vi "Main.vi"() -> ()   [LabVIEW 2019]
doc: "The myRIO Project template acquires acceleration data from the onboard accelerometer and displays the changes of acceleration values in a waveform chart."
uses:
  <vilib>/Platform/TimedLoop/XDataNode/timing_clust.ctl
  <vilib>/Platform/TimedLoop/XDataNode/nitl_modes.ctl
  <vilib>/Platform/TimedLoop/XDataNode/wakeup.ctl
  <vilib>/myRIO/Instrument Drivers/Onboard IO/AI/typedefs/AI Reference.ctl
  <vilib>/myRIO/Common/Instrument Driver Framework/Utilities/typedefs/myRIO Generic Hardware Reference.ctl
  <vilib>/myRIO/Common/Instrument Driver Framework/Utilities/typedefs/Hardware Version Enum.ctl
  <vilib>/myRIO/Common/Instrument Driver Framework/Utilities/typedefs/myRIO v1.0 Reference.ctl
  <vilib>/myRIO/Common/Instrument Driver Framework/Utilities/typedefs/Generic FPGA Reference.ctl
  <vilib>/myRIO/Common/Instrument Driver Framework/myRIO v1.0/AI/typedefs/AI Channels List.ctl
  <vilib>/myRIO/Common/Instrument Driver Framework/myRIO v1.0/AI/typedefs/AI Channels Enum.ctl
  <vilib>/myRIO/Common/Instrument Driver Framework/Utilities/typedefs/Analog Scaling Constants List.ctl
  <vilib>/myRIO/Common/Instrument Driver Framework/Utilities/typedefs/Analog Scaling Constants.ctl
  <vilib>/userDefined/High Color/nirio_resource_hc.ctl
  <vilib>/Simulation/Shared/_Datatypes/SIM SISO Transfer Function.ctl
  <vilib>/myRIO/Instrument Drivers/Onboard IO/AO/typedefs/AO Reference.ctl
  <vilib>/myRIO/Common/Instrument Driver Framework/myRIO v1.0/AO/typedefs/AO Channels List.ctl
  <vilib>/myRIO/Common/Instrument Driver Framework/myRIO v1.0/AO/typedefs/AO Channels Enum.ctl
  <vilib>/myRIO/Common/Instrument Driver Framework/Utilities/vis/Is FPGA Ref Available.vi
  <vilib>/myRIO/Common/Instrument Driver Framework/myRIO v1.0/AI/vis/myRIO v1.1 Open AI.vi
  <vilib>/myRIO/Instrument Drivers/Onboard IO/AI/vis/Read.vi
  <vilib>/Simulation/DiscreteLinear/Implementation/NILVSim Discrete Transfer Function Direct.llb/SIM Discrete Transfer Function Diagram (SISO).vi
  <vilib>/myRIO/Common/Instrument Driver Framework/myRIO v1.0/AO/vis/myRIO v1.1 Open AO.vi
  <vilib>/myRIO/Instrument Drivers/Onboard IO/AO/vis/Write.vi
  <vilib>/myRIO/Common/Instrument Driver Framework/Utilities/vis/Validate Channels.vi
  <vilib>/myRIO/Common/Instrument Driver Framework/myRIO v1.0/AI/vis/myRIO v1.0 Reserve AI.vi
  <vilib>/Simulation/ContinuousLinear/Implementation/Shared/SIM Transfer Function Support.llb/SIM TransferFunction Normalize to Buffer.vi
  <vilib>/Simulation/DiscreteLinear/Implementation/Shared/SIM Init Discrete States.vi
  <vilib>/Simulation/DiscreteLinear/Implementation/NILVSim Discrete Transfer Function Direct.llb/SIM Transfer Function Direct core (SISO).vi
  <vilib>/myRIO/Common/Instrument Driver Framework/myRIO v1.0/AO/vis/myRIO v1.0 Reserve AO.vi
  <vilib>/myRIO/Common/Instrument Driver Framework/myRIO v1.0/AI/vis/myRIO v1.0 Build MUX Configuration AI.vi
  <vilib>/myRIO/Common/Instrument Driver Framework/myRIO v1.0/Resource Manager/vis/myRIO v1.0 Reserve Channel List.vi
  <vilib>/Simulation/ContinuousLinear/Implementation/Shared/SIM Transfer Function Support.llb/SIM TransferFunction Normalize.vi
  <vilib>/myRIO/Common/Instrument Driver Framework/myRIO v1.0/AO/vis/myRIO v1.0 Build MUX Configuration AO.vi
  <vilib>/myRIO/Common/Instrument Driver Framework/myRIO v1.0/Resource Manager/vis/myRIO v1.0 Reserve Channel.vi
  <vilib>/myRIO/Common/Instrument Driver Framework/myRIO v1.0/Resource Manager/vis/myRIO v1.0 Unreserve Channel.vi
  <vilib>/Simulation/Implementation/Shared/SIM Polynomials.llb/SIM Remove Zero Coefficients (DBL).vi
  <vilib>/myRIO/Common/Instrument Driver Framework/myRIO v1.0/Resource Manager/vis/myRIO v1.0 Build Mutex Name.vi
  <vilib>/functionblocks/Counter/Pulse Timer/Pulse Timer.vi
  <vilib>/Utility/VariantDataType/GetNumericInfo.vi
  <vilib>/Utility/error.llb/Error Cluster From Error Code.vi
  <vilib>/myRIO/Common/Instrument Driver Framework/myRIO v1.0/myRIO v1.1 Open.vi
  <vilib>/myRIO/Common/Instrument Driver Framework/myRIO v1.0/AI/vis/myRIO v1.0 Get Scaling Constants AI.vi
  <vilib>/myRIO/Common/Instrument Driver Framework/Utilities/vis/IO Manager.vi
  <vilib>/myRIO/Common/Instrument Driver Framework/Utilities/vis/Configuration Manager.vi
  <vilib>/myRIO/Common/Instrument Driver Framework/myRIO v1.0/myRIO v1.0 Close.vi
  <vilib>/myRIO/Common/Instrument Driver Framework/myRIO v1.0/AI/vis/myRIO v1.0 Read AI.vi
  <vilib>/Simulation/Implementation/Shared/SIM Polynomials.llb/SIM Divide Polynomials (DBL).vi
  <vilib>/Simulation/Implementation/Shared/SIM BuildSimErr.vi
  <vilib>/myRIO/Common/Instrument Driver Framework/myRIO v1.0/AO/vis/myRIO v1.0 Get Scaling Constants AO.vi
  <vilib>/myRIO/Common/Instrument Driver Framework/myRIO v1.0/AO/vis/myRIO v1.0 Write AO.vi
  <vilib>/platform/TimedLoop/XDataNode/XDataNode.xnode
  <vilib>/functionblocks/FB Core/FB Core.xnode
  <vilib>/myRIO/Express VI/Onboard IO/AI/AI Express VI.xnode
  <vilib>/myRIO/Instrument Drivers/Onboard IO/AI/vis/myRIO AI Open.xnode
  <vilib>/Simulation/Implementation/XNodeFramework/SimXNode/SimX.xnode
  <vilib>/myRIO/Express VI/Onboard IO/AO/AO Express VI.xnode
  <vilib>/myRIO/Instrument Drivers/Onboard IO/AO/vis/myRIO AO Open.xnode
  <vilib>/Platform/TimedLoop/XDataNode/XDNodeRunTimeDep.lvlib
  <vilib>/myRIO/Instrument Drivers/Onboard IO/AI/AI.lvlib
  <vilib>/myRIO/Instrument Drivers/Onboard IO/AO/AO.lvlib
  <vilib>/functionblocks/NI_FunctionBlock Libraries.lvlib
panel:
  out "frequecy":dbl(graph)=-0.0 caption="interrupt frequency"
  in  "interrupt time(ms)":i32=1000
  in  "Interrupt":bool
  out "sine wave":dbl(graph)=-0.0 caption="Interrupt"
  out "x[um]":dbl(graph)=2.4390249999999867
  in  "initialize z":bool
  out "right[V]":dbl=-0.00025
  out "left[V]":dbl=-0.00025
  in  "Stop EM":bool=TRUE
  out "Current Output EM":dbl(graph)=-0.0
  out "Error":errorcluster
  in  "Stop":bool
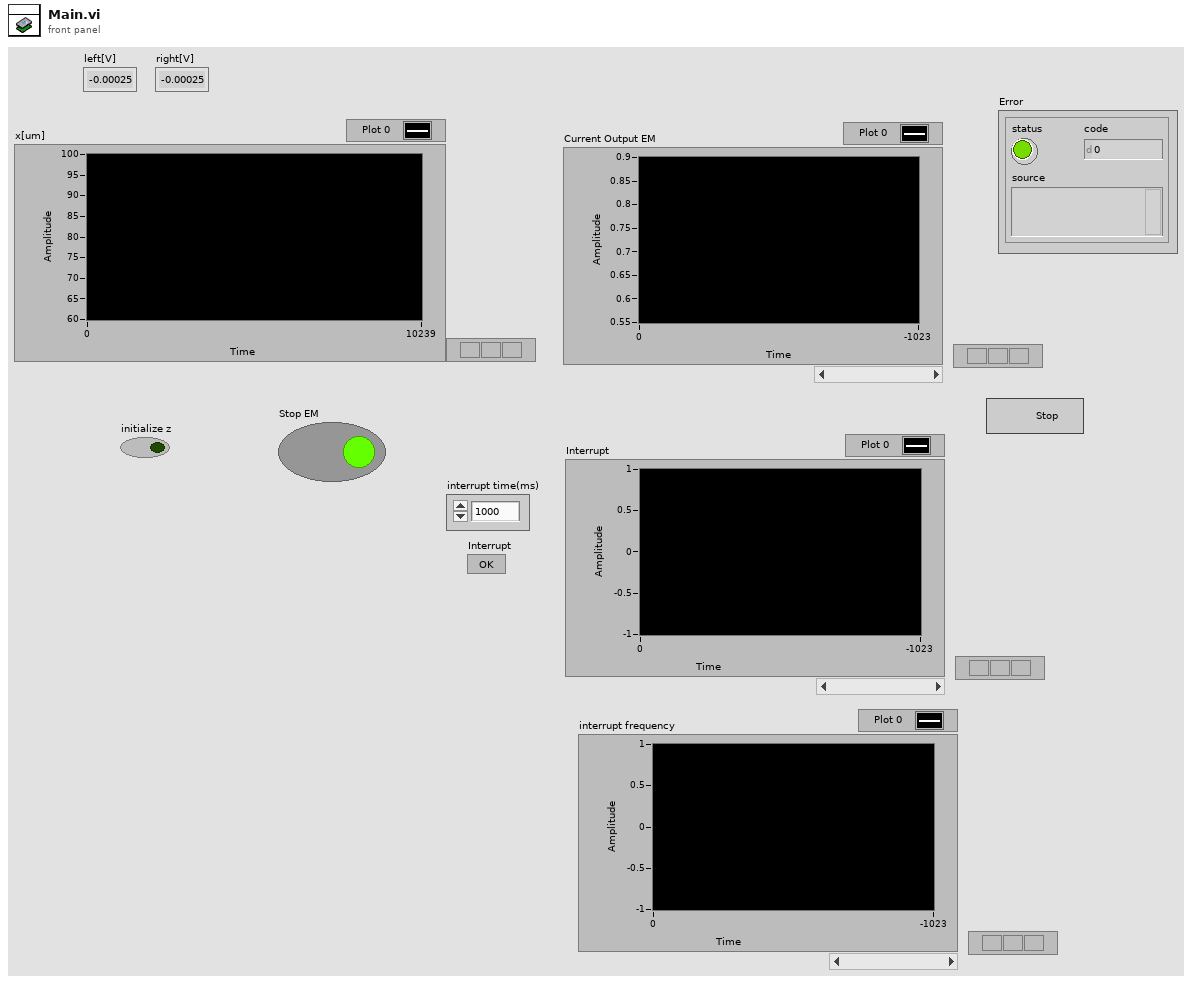
[diagram p1: front panel]
types:
  T1 = typedef "SIM SISO Transfer Function.ctl" = cluster{"Numerator":dbl[], "Denominator":dbl[]}
  T2 = typedef "AO.lvlib/AO Reference.ctl" = cluster{"myRIO Reference":T3, "AO Channel List":T7, "AO Scaling Constant List":T9}
  T3 = typedef "myRIO Generic Hardware Reference.ctl" = cluster{"myRIO Model":T4, "myRIO Hardware Reference":T5}
  T4 = typedef "Hardware Version Enum.ctl" = enum16{"Unknown", "myRIO-1900", "myRIO-1950", "roboRIO", "NI ELVIS RIO CM", "ELVIS III"}
  T5 = typedef "myRIO v1.0 Reference.ctl" = cluster{"Generic FPGA Reference":T6, "Allow multiple opens":bool}
  T6 = typedef "Generic FPGA Reference.ctl" = refnum<k20>
  T7 = typedef "AO Channels List.ctl" = T8[]
  T8 = typedef "AO Channels Enum.ctl" = enum16{"Not Connected", "AudioOut/Left", "AudioOut/Right", "C/AO0", "C/AO1", "A/AO0", "A/AO1", "B/AO0", "B/AO1"}
  T9 = typedef "Analog Scaling Constants List.ctl" = T10[]
  T10 = typedef "Analog Scaling Constants.ctl" = cluster{"LSB Weight (Volts)":dbl, "Offset (Volts)":dbl, "Signed?":bool}
  T11 = typedef "nirio_resource_hc.ctl" = tag
  T12 = typedef "AI.lvlib/AI Reference.ctl" = cluster{"myRIO Reference":T3, "AI Channels List":T13, "AI Scaling Constants List":T9}
  T13 = typedef "AI Channels List.ctl" = T14[]
  T14 = typedef "AI Channels Enum.ctl" = enum16{"Not Connected", "AudioIn/Left", "AudioIn/Right", "C/AI0", "C/AI1", "A/AI0", "A/AI1", "A/AI2", "A/AI3", "A/AI4", "A/AI5", "A/AI6", "A/AI7", "B/AI0", "B/AI1", "B/AI2", "B/AI3", "B/AI4", "B/AI5", "B/AI6", "B/AI7", "AI/AI0", "AI/AI1", "AI/AI2", "AI/AI3", "A/AI0 (DIFF)", "A/AI1 (DIFF)", "A/AI2 (DIFF)", "A/AI3 (DIFF)", "B/AI0 (DIFF)", "B/AI1 (DIFF)", "B/AI2 (DIFF)", "B/AI3 (DIFF)"}
  T15 = typedef "XDNodeRunTimeDep.lvlib/timing_clust.ctl" = cluster{"Expected End [f-1]":u64, "Actual End [f-1]":u64, "Finished Late? [f-1]":bool, "Expected End [i-1]":u64, "Actual End [i-1]":u64, "Finished Late? [i-1]":bool, "Expected Start [i]":u64, "Actual Start [i]":u64, "Expected Start [f]":u64, "Actual Start [f]":u64, "Source Name":string, "Structure Name":string, "Period":i64, "Deadline":i64, "Offset":i64, "Start":i64, "Priority":i32, "Timeout":i32, "Mode":T16, "Wakeup Reason":T17, "Error":errorcluster, "Source Type":string, "Secondary Source Type":string, "Global End Time":u64, "Global Start Time":u64, "Frame Duration":u64, "Iteration Duration":u64, "Assigned CPU":i32, "I/O Scan Engine Mode":u32}
  T16 = typedef "XDNodeRunTimeDep.lvlib/nitl_modes.ctl" = enum32{"No Change", "Process missed periods, maintain original phase", "Discard missed periods, maintain original phase", "Process missed periods, ignore original phase", "Discard missed periods, ignore original phase"}
  T17 = typedef "XDNodeRunTimeDep.lvlib/wakeup.ctl" = enum32{"Normal", "Aborted", "Asynchronous wakeup", "Timing source error", "Timed loop error", "Timeout"}
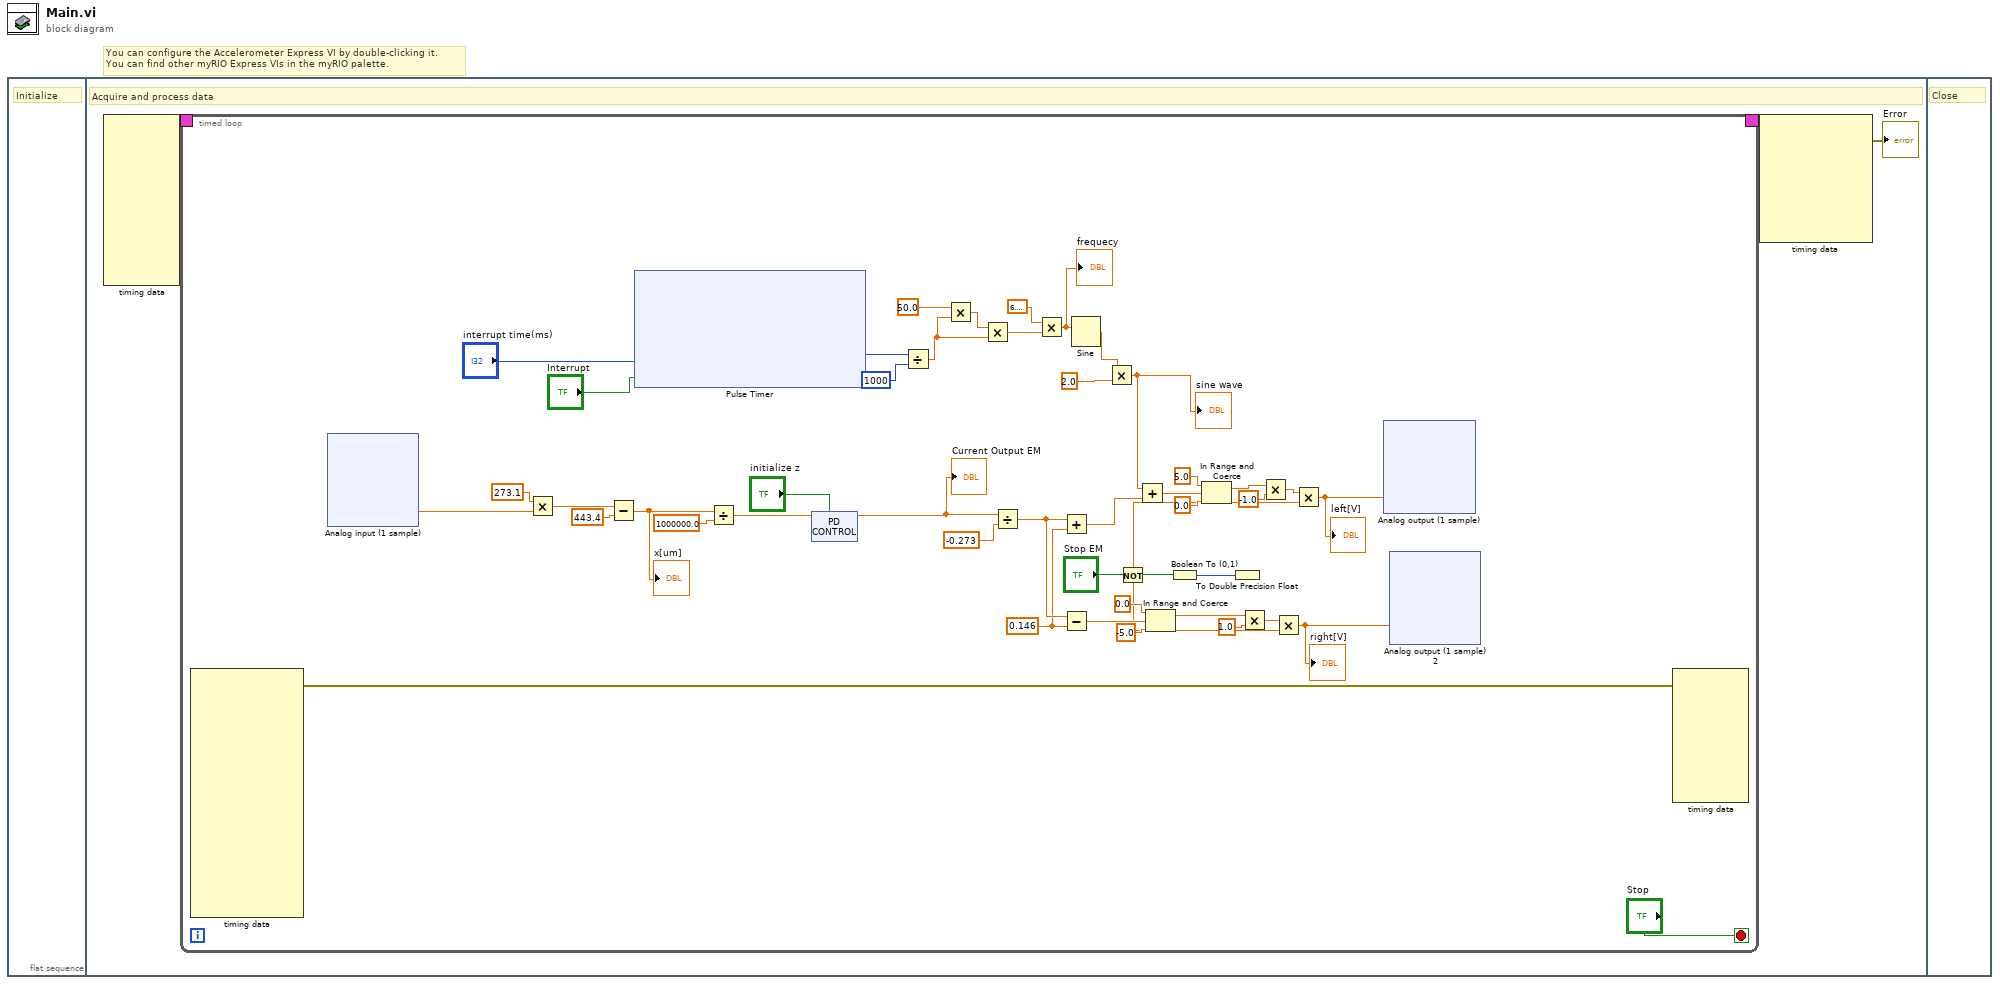
[diagram p0: block diagram]
diagram:
  # "You can configure the Accelerometer Express VI by double-clicking it.\nYou can find other myRIO Express VIs in the myRIO palette."
  n1 = flat-sequence {
    frame #0 {
      # "Initialize"
    }
    frame #1 {
      # "Acquire and process data"
      n2 = node-c288() -> (w3:T15)  [unwired: 10 in]
      n3 = timed-loop {
        timing: w3 -> [_]
        timing-out: [_] -> w2
        stop <- "Stop" stop-if-true
        w33 = 0.146 ("y")
        n4 = node-c288() -> (w48:errorcluster)  [unwired: 1 in, 15 out]
        n5 = xnode "Analog input (1 sample)"() -> ("C/AI1 (AI1)"=w23:dbl)  [unwired: 1 in, 1 out]
        n6 = Multiply(x=273.1, y=w23) -> (x*y=w20:dbl)
        n7 = Subtract(x=w20, y=443.4 ("x")) -> (x-y=w19:dbl)
        "x[um]" <- w19
        n8 = xnode "Pulse Timer"("preset time (ms)"="interrupt time(ms)", "input"="Interrupt") -> ("elapsed time (ms)"=w9:i32)  [unwired: 1 in, 2 out]
        n9 = Divide(x=w19, y=1000000.0) -> (x/y=w28:dbl)
        n10 = xnode "PD CONTROL"("input u(k)"=w28, "initialize"="initialize z") -> ("output y(k)"=w24:dbl)  [unwired: 1 in, 1 out]
        "Current Output EM" <- w24
        n11 = Divide(x=w9, y=1000) -> (x/y=w5:dbl)
        n12 = Multiply(x=50.0 ("y"), y=w5) -> (x*y=w7:dbl)
        n13 = Multiply(x=w7, y=w5) -> (x*y=w12:dbl)
        n14 = Divide(x=w24, y=-0.273) -> (x/y=w34:dbl)
        n15 = Multiply(x=6.283185307179586, y=w12) -> (x*y=w4:dbl)
        "frequecy" <- w4
        n16 = Add(x=w34, y=w33) -> (x+y=w17:dbl)
        n17 = Subtract(x=w34, y=w33) -> (x-y=w35:dbl)
        n18 = Sine(x=w4) -> (sin(x)=w16:dbl)
        n19 = Multiply(x=w16, y=2.0) -> (x*y=w14:dbl)
        "sine wave" <- w14
        n20 = Not(x="Stop EM") -> (.not. x?=w36:bool)
        n21 = Add(x=w14, y=w17) -> (x+y=w18:dbl)
        n22 = In Range and Coerce(upper limit=0.0 ("x"), x=w35, lower limit=-5.0) -> (coerced(x)=w41:dbl)  [unwired: 1 out]
        n23 = Boolean To (0,1)(Boolean=w36) -> (0, 1=w38:i16)
        n24 = In Range and Coerce(upper limit=5.0 ("x"), x=w18, lower limit=0.0) -> (coerced(x)=w25:dbl)  [unwired: 1 out]
        n25 = To Double Precision Float(number=w38) -> (double precision float=w30:dbl)
        n26 = Multiply(x=w41, y=1.0) -> (x*y=w31:dbl)
        n27 = Multiply(x=w25, y=-1.0) -> (x*y=w32:dbl)
        n28 = Multiply(x=w31, y=w30) -> (x*y=w26:dbl)
        "right[V]" <- w26
        n29 = Multiply(x=w32, y=w30) -> (x*y=w27:dbl)
        "left[V]" <- w27
        n30 = xnode "Analog output (1 sample)"("C/AO0 (AO0)"=w27) -> ()  [unwired: 1 in, 1 out]
        n31 = xnode "Analog output (1 sample) 2"("C/AO1 (AO1)"=w26) -> ()  [unwired: 1 in, 1 out]
        n32 = node-c288(w48) -> ()  [unwired: 7 in, 1 out]
      }
      n33 = node-c288(w2) -> (→"Error":errorcluster)  [unwired: 6 out]
    }
    frame #2 {
      # "Close"
    }
  }
